vi "Kolor dynamicznie.vi"(8 "error in (no error)":errorcluster, 10 "Data":T1, 11 "WaveformChart in":refnum<vi>) -> (0 "error out":errorcluster)   [LabVIEW 2013]
doc: "Zmienia kolor pierwszego wykresu\nw przypadku przekroczenia zakresów.\n- Zmienia kolory punktów!"
uses:
  inne pliki/Data.ctl
  inne pliki/Params.ctl
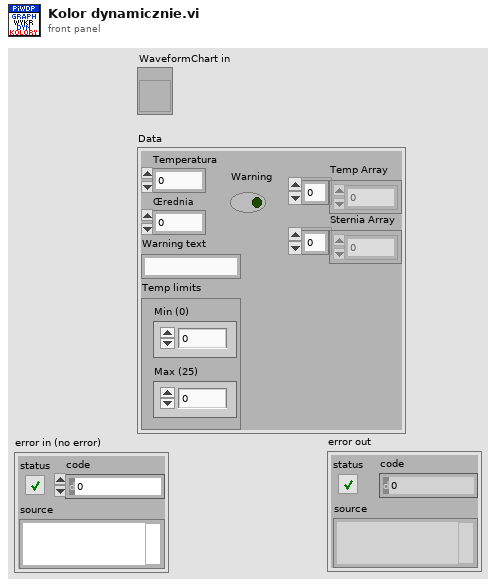
[diagram p1: front panel]
types:
  T1 = typedef "Data.ctl" = cluster{"Temperatura":dbl, "Œrednia":dbl, "Warning":bool, "Warning text ":string, "Temp limits":T2, "Temp Array":dbl[], "Sternia Array":dbl[]}
  T2 = typedef "Params.ctl" = cluster{"Max (25)":dbl, "Min (0)":dbl}
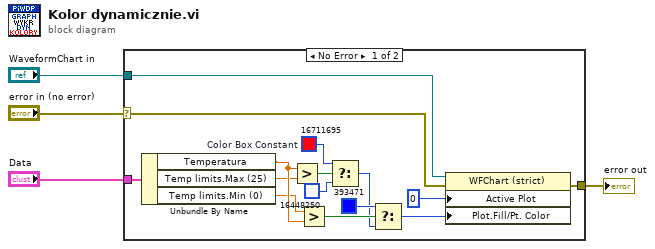
[diagram p0: block diagram]
diagram:
  n1 = case shown="No Error" "error in (no error)" {
    selector: "error in (no error)" -> [w5 w20]
    tunnel: "Data" -> [w9 _]
    tunnel: "WaveformChart in" -> [w7 _]
    tunnel: [w6 w20] -> w2
    frame No Error {
      w16 = u32 16711695  # Color Box Constant
      n2 = Unbundle By Name(w9) -> ("Temperatura"=w19:dbl, "Temp limits.Max (25)"=w11:dbl, "Temp limits.Min (0)"=w12:dbl)
      n3 = Greater?(x=w19, y=w11) -> (0:w10:bool)
      n4 = Greater?(x=w12, y=w19) -> (0:w15:bool)
      n5 = Select(t=w16, s=w10, f=u32 16448250) -> (s? t:f=w14:u32)
      n6 = Select(t=u32 393471, s=w15, f=w14) -> (s? t:f=w17:u32)
      n7 = property on="Property Node" class="WFChart (strict)"(reference=w7, error in=w5, "Active Plot"=u32 0, "Plot.Fill/Pt. Color"=w17) -> (error out=w6:errorcluster)  [unwired: 1 out]
    }
    frame Error {
    }
  }
  "error out" <- w2
